vi "NistCSV2Cluster.vi"(8 "error in (no error)":errorcluster, 11 "NISTPath":path) -> (0 "error out":errorcluster, 2 "NISTData":T1 {"DataAnlysisArray"."TimeStamp" format="%^<%.3X\n%x>T"; "DUTDataArray"."Time Stamp" format="%^<%.3X\n%x>T"; "NIDataArray"."Time Stamp" format="%^<%.3X\n%x>T"})   [LabVIEW 2014]
uses:
  typedefs/NIData.ctl
  typedefs/PhasorRectangular.ctl
  typedefs/DUTData.ctl
  typedefs/NISTData.ctl
  typedefs/NIDataArray.ctl
  typedefs/NICalcAnalysis.ctl
  typedefs/CalcPhasorError.ctl
  <vilib>/Utility/miscctls.llb/LVDateTimeRec.ctl
  <vilib>/Utility/file.llb/Read From Spreadsheet File (string).vi
panel:
  in  "NICalcAnalysis":T6 {"TimeStamp" format="%^<%.3X\n%x>T"}
  in  "DUTDataCluster":T5 {"Time Stamp" format="%^<%.3X\n%x>T"}
  in  "NIDataCluster":T3 {"Time Stamp" format="%^<%.3X\n%x>T"}
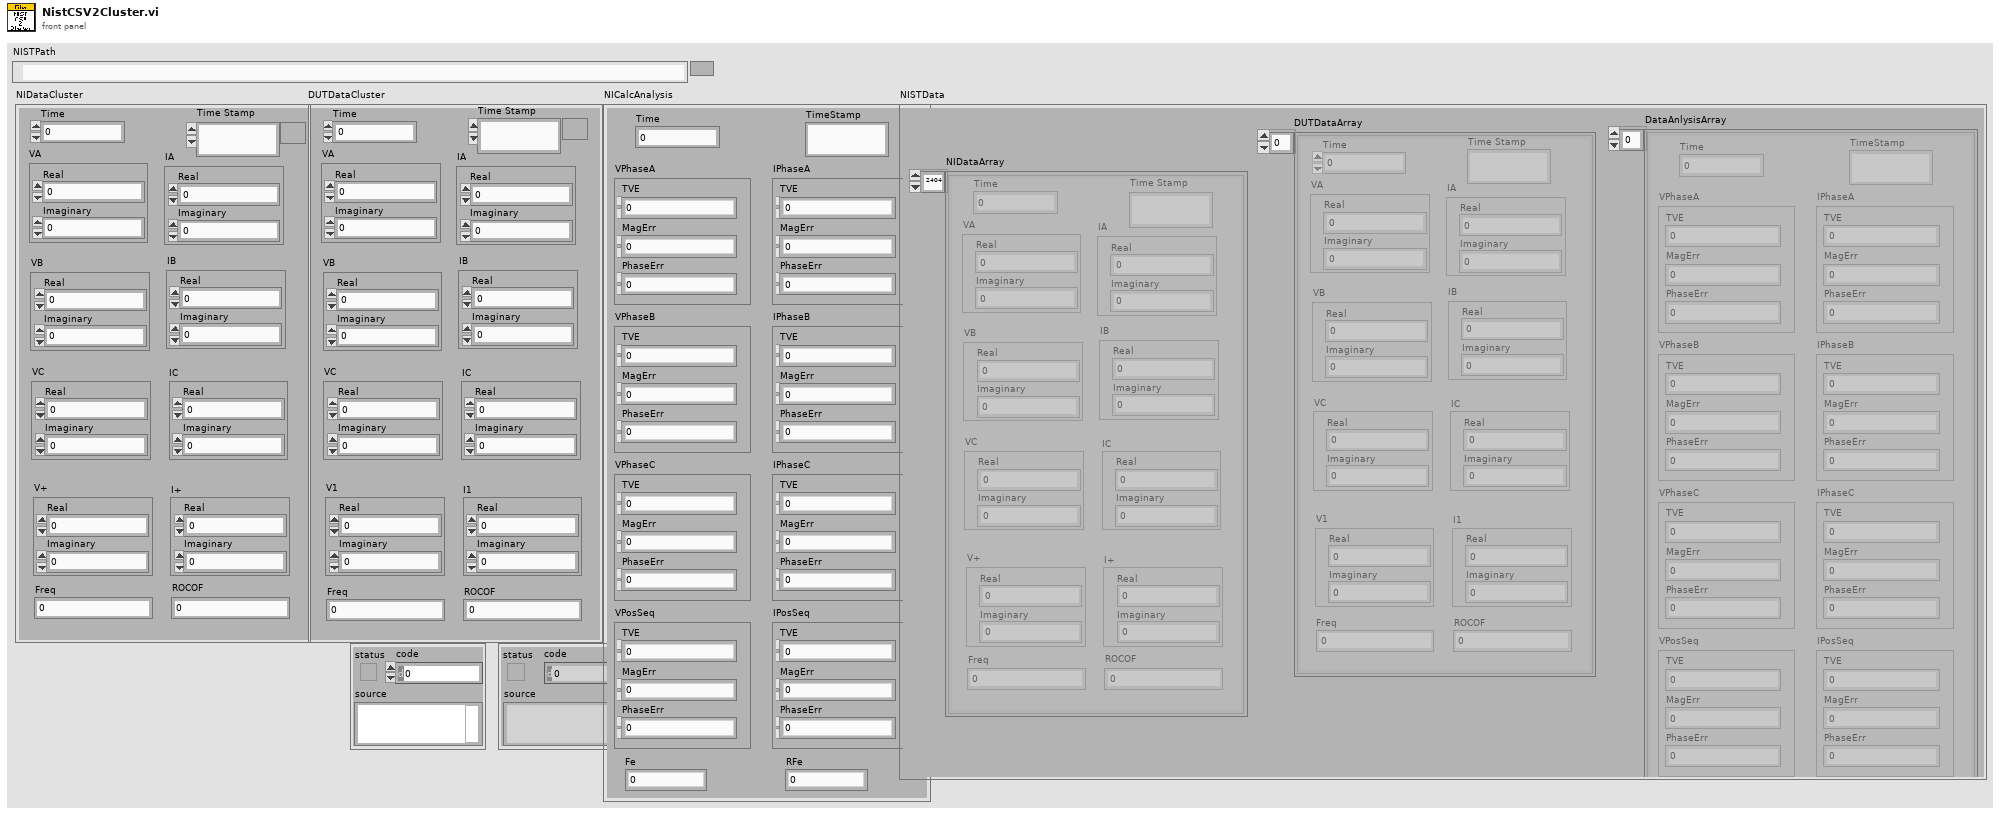
[diagram p1: front panel]
types:
  T1 = typedef "NISTData.ctl" = cluster{"NIDataArray":T2, "DUTDataArray":T5[], "DataAnlysisArray":T6[]}
  T2 = typedef "NIDataArray.ctl" = T3[]
  T3 = typedef "NIData.ctl" = cluster{"Time":dbl, "VA":T4, "VB":T4, "VC":T4, "V+":T4, "IA":T4, "IB":T4, "IC":T4, "I+":T4, "Freq":dbl, "ROCOF":dbl, "Time Stamp":timestamp}
  T4 = typedef "PhasorRectangular.ctl" = cluster{"Real":dbl, "Imaginary":dbl}
  T5 = typedef "DUTData.ctl" = cluster{"Time":dbl, "VA":T4, "VB":T4, "VC":T4, "V1":T4, "IA":T4, "IB":T4, "IC":T4, "I1":T4, "Freq":dbl, "ROCOF":dbl, "Time Stamp":timestamp}
  T6 = typedef "NICalcAnalysis.ctl" = cluster{"Time":dbl, "VPhaseA":T7, "IPhaseA":T7, "VPhaseB":T7, "IPhaseB":T7, "VPhaseC":T7, "IPhaseC":T7, "VPosSeq":T7, "IPosSeq":T7, "Fe":dbl, "RFe":dbl, "TimeStamp":timestamp}
  T7 = typedef "CalcPhasorError.ctl" = cluster{"TVE":dbl, "MagErr":dbl, "PhaseErr":dbl}
  T8 = typedef "LVDateTimeRec.ctl" = cluster{"fractional second":dbl, "second":i32, "minute":i32, "hour":i32, "day of month":i32, "month":i32, "year":i32, "day of week":i32, "day of year":i32, "DST":i32}
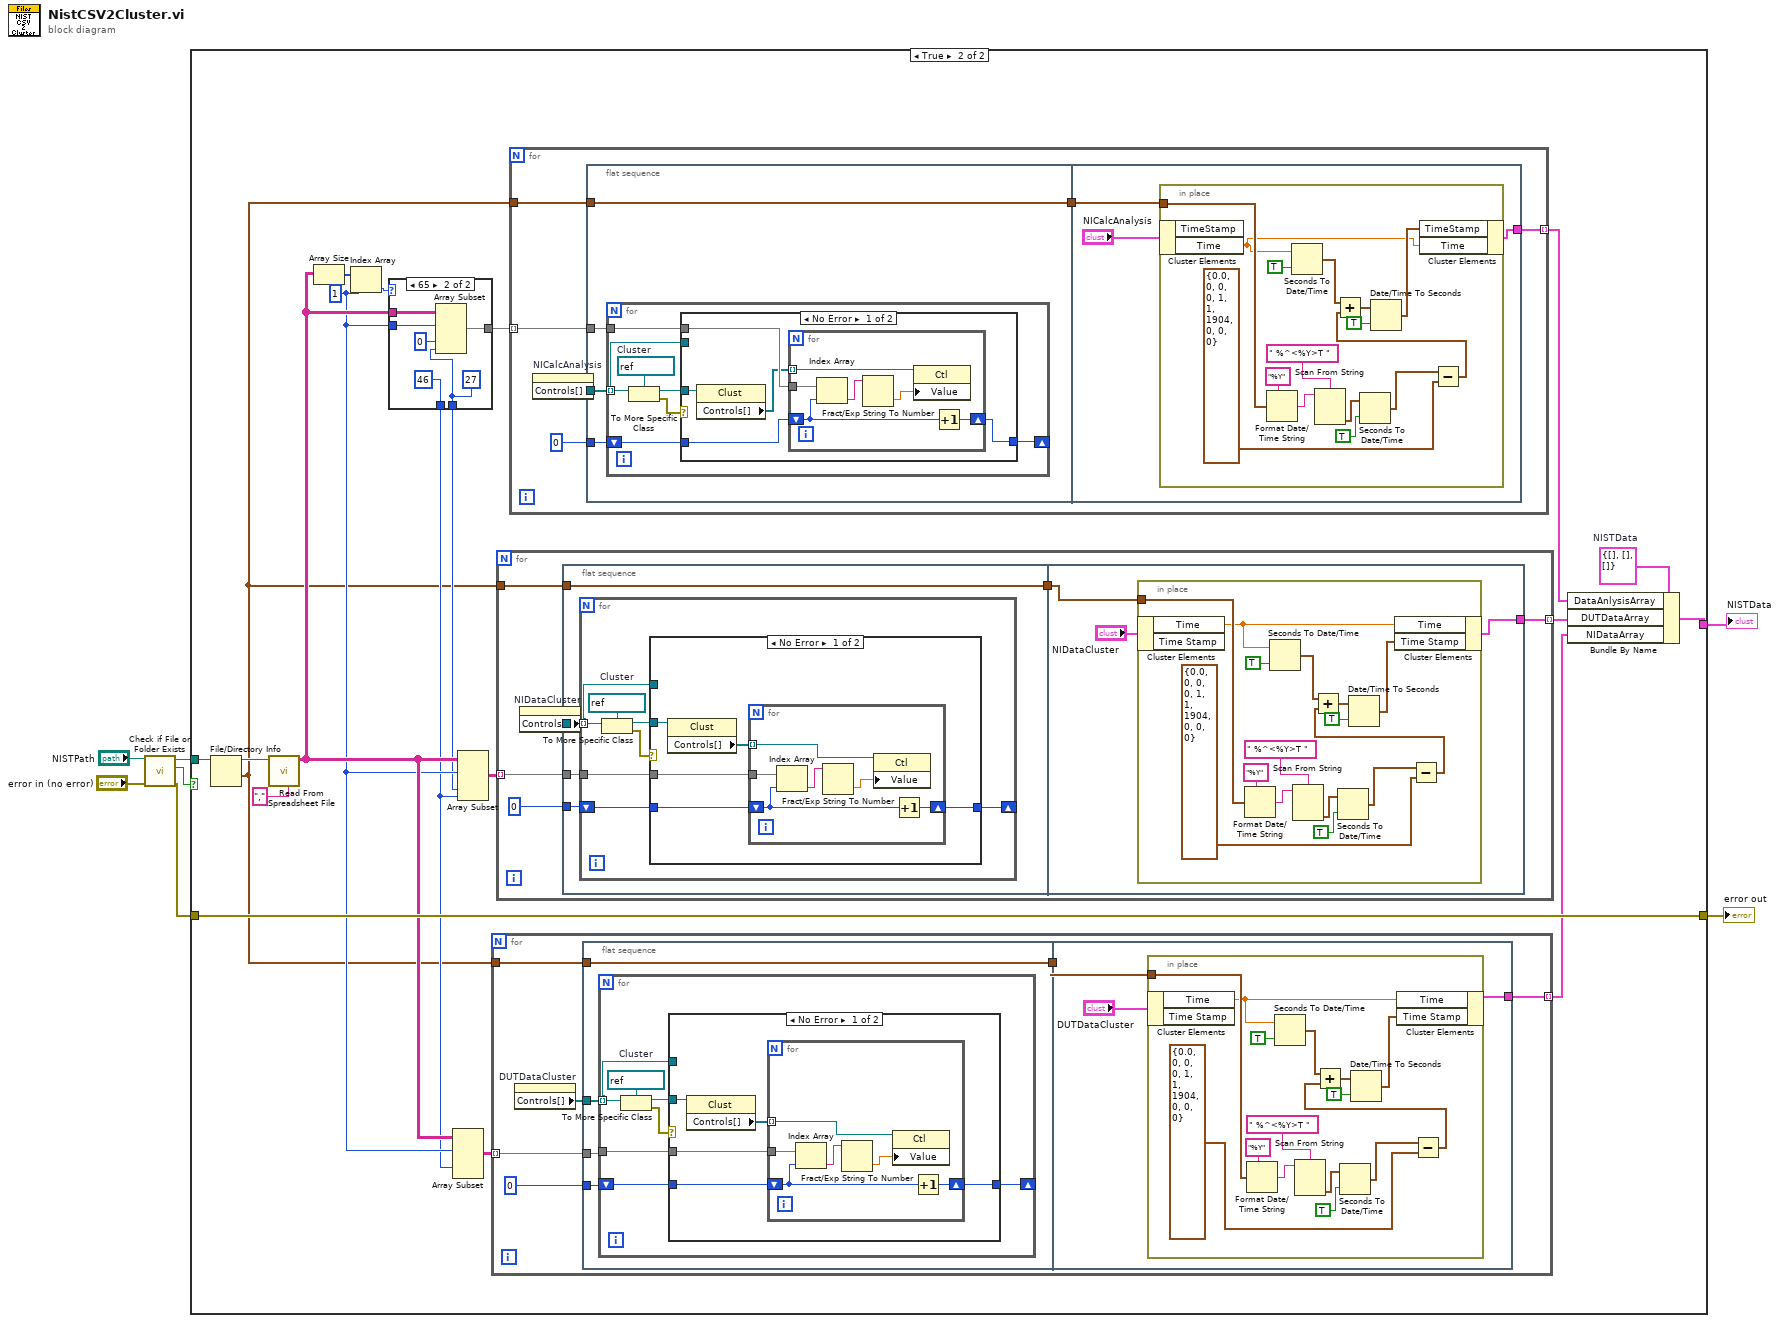
[diagram p0: block diagram]
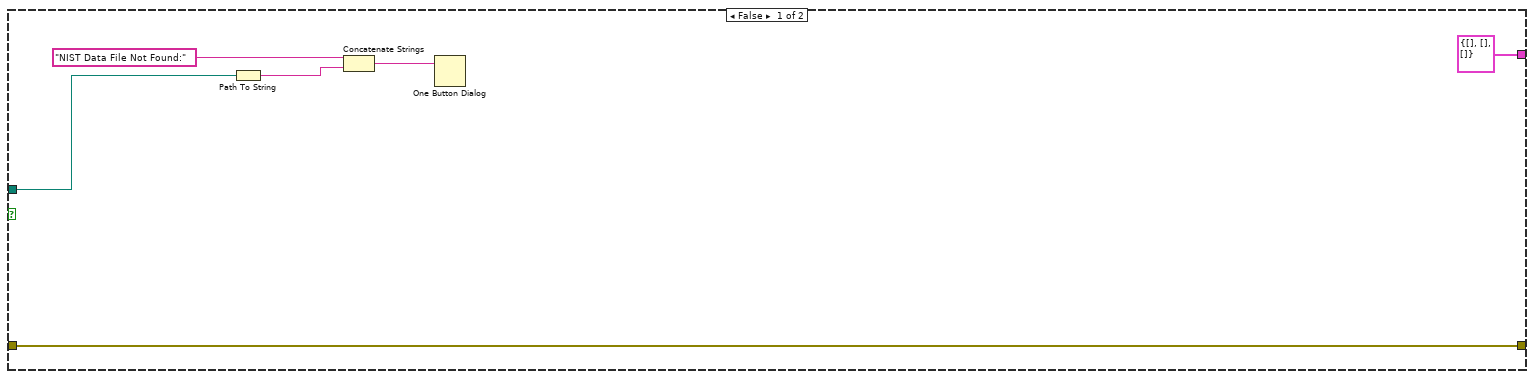
[diagram p2: hidden frame]
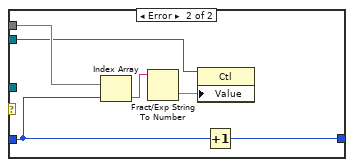
[diagram p3: hidden frame]
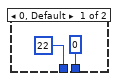
[diagram p4: hidden frame]
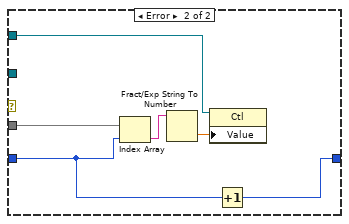
[diagram p5: hidden frame]
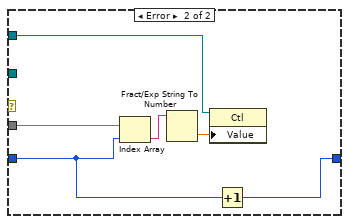
[diagram p6: hidden frame]
diagram:
  n1 = call <vilib>:"Check if File or Folder Exists.vi"("error in (no error)"="error in (no error)", "path"="NISTPath") -> ("error out"=w3:errorcluster, "file or folder exists?"=w4:bool, "dup path"=w5:path)  [unwired: 7 in]
  n2 = case shown="True" w4 {
    tunnel: w5 -> [w11 w32]
    tunnel: w3 -> [w9 w28]
    tunnel: [w9 w28] -> w2
    tunnel: [T1 {"NIDataArray"=[], "DUTDataArray"=[], "DataAnlysisArray"=[]} ("NISTData") w19] -> w1
    frame False {
      n3 = Path To String(path=w11) -> (string=w12:string)
      n4 = Concatenate Strings("NIST Data File Not Found:", w12) -> (w10:string)
      n5 = One Button Dialog(message=w10) -> ()  [unwired: 1 in, 1 out]
    }
    frame True {
      w22 = 1 ("index")
      w27 = T1 {"NIDataArray"=[], "DUTDataArray"=[], "DataAnlysisArray"=[]}  # NISTData
      n6 = File/Directory Info(path=w32) -> (path out=w26:path, last mod=w15:timestamp)  [unwired: 1 in, 5 out]
      n7 = call-poly <vilib>:"Read From Spreadsheet File.vi"("delimiter (\\t)"="," ("delimiter (\\t)"), "file path (dialog if empty)"=w26) -> ("all rows"=w23:string[][])  [unwired: 5 in, 4 out]
      n8 = Array Size(array=w23) -> (size(s)=w25:i32[])
      n9 = Index Array(array=w25, index=w22) -> (element=w24:i32)
      n10 = case shown="65" w24 {
        tunnel: w23 -> [_ w92]
        tunnel: w22 -> [_ w91]
        tunnel: [0 ("index") w88] -> w21
        tunnel: [22 ("length") 46 ("length")] -> w20
        tunnel: [_ w87] -> w16
        frame 0, Default {
        }
        frame 65 {
          w88 = 27 ("index")
          n11 = Array Subset(array=w92, index (row)=w91, index (col)=0 ("index"), length (col)=w88) -> (w87:string[][])  [unwired: 1 in]
        }
      }
      n12 = Array Subset(array=w23, index (row)=w22, index (col)=w20) -> (w29:string[][])  [unwired: 2 in]
      n13 = Array Subset(array=w23, index (row)=w22, index (col)=w21, length (col)=w20) -> (w30:string[][])  [unwired: 1 in]
      n14 = for {
        tunnel: w29 -> [w98] mode=indexing
        tunnel: [w93] -> w17 mode=indexing
        tunnel: w15 -> [w95]
        n15 = property on="DUTDataCluster" class="Clust (strict)"() -> ("Controls[]"=w96:refnum<vi>[])  [unwired: 2 in, 2 out]
        n16 = flat-sequence {
          tunnel: w98 -> [w102]
          tunnel: 0 ("index") -> [w101]
          tunnel: w96 -> [w100]
          tunnel: w95 -> [w99]
          tunnel: [w99] -> w94
          tunnel: w94 -> [w128]
          tunnel: [w127] -> w93
          frame #0 {
            n17 = for {
              tunnel: w100 -> [w103] mode=indexing
              tunnel: w102 -> [w106]
              shift-right: [w104] -> _
              shift-left: w101 -> [w105]
              w109 = refnum<vi> refnum  # Cluster
              n18 = To More Specific Class(target class=w109, reference=w103) -> (specific class reference=w107:refnum<vi>, error out=w108:errorcluster)  [unwired: 1 in]
              n19 = case shown="No Error" w108 {
                tunnel: w107 -> [w114 _]
                tunnel: w106 -> [w112 w126]
                tunnel: w105 -> [w111 w125]
                tunnel: [w110 w124] -> w104
                tunnel: w103 -> [_ w121]
                frame No Error {
                  n20 = property class="Clust"(reference=w114) -> ("Controls[]"=w113:refnum<vi>[])  [unwired: 1 in, 2 out]
                  n21 = for {
                    tunnel: w113 -> [w117] mode=indexing
                    tunnel: w112 -> [w120]
                    shift-right: [w115] -> w110
                    shift-left: w111 -> [w119]
                    n22 = Index Array(array=w120, index=w119) -> (element=w118:string)
                    n23 = Fract/Exp String To Number(string=w118) -> (number=w116:dbl)  [unwired: 3 in, 1 out]
                    n24 = property class="Ctl"(reference=w117, "Value"=w116) -> ()  [unwired: 1 in, 2 out]
                    n25 = Increment(x=w119) -> (x+1=w115:i32)
                  }
                }
                frame Error {
                  n26 = Index Array(array=w126, index=w125) -> (element=w123:string)
                  n27 = Fract/Exp String To Number(string=w123) -> (number=w122:dbl)  [unwired: 3 in, 1 out]
                  n28 = property class="Ctl"(reference=w121, "Value"=w122) -> ()  [unwired: 1 in, 2 out]
                  n29 = Increment(x=w125) -> (x+1=w124:i32)
                }
              }
            }
          }
          frame #1 {
            n30 = in-place {
              in-place-border: w128 -> [w144]
              n31 = in-place-cluster #1("DUTDataCluster") -> ("Time"=w140:dbl)  [unwired: 1 out]
              n32 = Format Date/Time String(time format string (%c)="%Y", seconds (now)=w144) -> (date/time string=w141:string)  [unwired: 1 in]
              n33 = Seconds To Date/Time(time stamp (now)=w140, to UTC (F)=TRUE) -> (date time rec=w138:T8)
              n34 = Scan From String(format string=" %^<%Y>T ", input string=w141) -> (output 1=w139:timestamp)  [unwired: 3 in, 3 out]
              n35 = Seconds To Date/Time(time stamp (now)=w139, to UTC (F)=TRUE ("is UTC (F)")) -> (date time rec=w135:T8)
              n36 = Subtract(x=w135, y=T8 {"fractional second"=0.0, "second"=0, "minute"=0, "hour"=0, "day of month"=1, "month"=1, "year"=1904, "day of week"=0, "day of year"=0, "DST"=0}) -> (x-y=w134:T8)
              n37 = Add(x=w138, y=w134) -> (x+y=w137:T8)
              n38 = Date/Time To Seconds(1:TRUE ("is UTC (F)"), 2:w137) -> (0:w136:timestamp)
              n39 = in-place-cluster #1("Time"=w140, "Time Stamp"=w136) -> (w127:T5)
            }
          }
        }
      }
      n40 = for {
        tunnel: w30 -> [w150] mode=indexing
        tunnel: [w145] -> w18 mode=indexing
        tunnel: w15 -> [w146]
        n41 = property on="NIDataCluster" class="Clust (strict)"() -> ("Controls[]"=w148:refnum<vi>[])  [unwired: 2 in, 2 out]
        n42 = flat-sequence {
          tunnel: w150 -> [w154]
          tunnel: 0 ("index") -> [w153]
          tunnel: w148 -> [w152]
          tunnel: [w151] -> w147
          tunnel: w146 -> [w151]
          tunnel: w147 -> [w180]
          tunnel: [w179] -> w145
          frame #0 {
            n43 = for {
              tunnel: w152 -> [w155] mode=indexing
              tunnel: w154 -> [w158]
              shift-right: [w156] -> _
              shift-left: w153 -> [w157]
              w161 = refnum<vi> refnum  # Cluster
              n44 = To More Specific Class(target class=w161, reference=w155) -> (specific class reference=w159:refnum<vi>, error out=w160:errorcluster)  [unwired: 1 in]
              n45 = case shown="No Error" w160 {
                tunnel: w159 -> [w166 _]
                tunnel: w158 -> [w164 w178]
                tunnel: w157 -> [w163 w177]
                tunnel: [w162 w176] -> w156
                tunnel: w155 -> [_ w173]
                frame No Error {
                  n46 = property class="Clust"(reference=w166) -> ("Controls[]"=w165:refnum<vi>[])  [unwired: 1 in, 2 out]
                  n47 = for {
                    tunnel: w165 -> [w169] mode=indexing
                    tunnel: w164 -> [w172]
                    shift-right: [w167] -> w162
                    shift-left: w163 -> [w171]
                    n48 = Index Array(array=w172, index=w171) -> (element=w170:string)
                    n49 = Fract/Exp String To Number(string=w170) -> (number=w168:dbl)  [unwired: 3 in, 1 out]
                    n50 = property class="Ctl"(reference=w169, "Value"=w168) -> ()  [unwired: 1 in, 2 out]
                    n51 = Increment(x=w171) -> (x+1=w167:i32)
                  }
                }
                frame Error {
                  n52 = Index Array(array=w178, index=w177) -> (element=w175:string)
                  n53 = Fract/Exp String To Number(string=w175) -> (number=w174:dbl)  [unwired: 3 in, 1 out]
                  n54 = property class="Ctl"(reference=w173, "Value"=w174) -> ()  [unwired: 1 in, 2 out]
                  n55 = Increment(x=w177) -> (x+1=w176:i32)
                }
              }
            }
          }
          frame #1 {
            n56 = in-place {
              in-place-border: w180 -> [w196]
              n57 = in-place-cluster #2("NIDataCluster") -> ("Time"=w192:dbl)  [unwired: 1 out]
              n58 = Format Date/Time String(time format string (%c)="%Y", seconds (now)=w196) -> (date/time string=w193:string)  [unwired: 1 in]
              n59 = Seconds To Date/Time(time stamp (now)=w192, to UTC (F)=TRUE) -> (date time rec=w190:T8)
              n60 = Scan From String(format string=" %^<%Y>T ", input string=w193) -> (output 1=w191:timestamp)  [unwired: 3 in, 3 out]
              n61 = Seconds To Date/Time(time stamp (now)=w191, to UTC (F)=TRUE) -> (date time rec=w187:T8)
              n62 = Subtract(x=w187, y=T8 {"fractional second"=0.0, "second"=0, "minute"=0, "hour"=0, "day of month"=1, "month"=1, "year"=1904, "day of week"=0, "day of year"=0, "DST"=0}) -> (x-y=w184:T8)
              n63 = Add(x=w190, y=w184) -> (x+y=w189:T8)
              n64 = Date/Time To Seconds(1:TRUE ("is UTC (F)"), 2:w189) -> (0:w188:timestamp)
              n65 = in-place-cluster #2("Time"=w192, "Time Stamp"=w188) -> (w179:T3)
            }
          }
        }
      }
      n66 = for {
        tunnel: w16 -> [w37] mode=indexing
        tunnel: w15 -> [w36]
        tunnel: [w33] -> w14 mode=indexing
        n67 = property on="NICalcAnalysis" class="Clust (strict)"() -> ("Controls[]"=w34:refnum<vi>[])  [unwired: 2 in, 2 out]
        n68 = flat-sequence {
          tunnel: w34 -> [w42]
          tunnel: 0 ("index") -> [w41]
          tunnel: w37 -> [w40]
          tunnel: w36 -> [w39]
          tunnel: [w39] -> w35
          tunnel: w35 -> [w68]
          tunnel: [w67] -> w33
          frame #0 {
            n69 = for {
              tunnel: w42 -> [w43] mode=indexing
              shift-right: [w44] -> _
              shift-left: w41 -> [w46]
              tunnel: w40 -> [w45]
              w49 = refnum<vi> refnum  # Cluster
              n70 = To More Specific Class(target class=w49, reference=w43) -> (specific class reference=w47:refnum<vi>, error out=w48:errorcluster)  [unwired: 1 in]
              n71 = case shown="No Error" w48 {
                tunnel: w47 -> [w54 _]
                tunnel: w46 -> [w53 w63]
                tunnel: w45 -> [w51 w64]
                tunnel: [w52 w62] -> w44
                tunnel: w43 -> [_ w61]
                frame No Error {
                  n72 = property class="Clust"(reference=w54) -> ("Controls[]"=w50:refnum<vi>[])  [unwired: 1 in, 2 out]
                  n73 = for {
                    tunnel: w50 -> [w57] mode=indexing
                    tunnel: w51 -> [w60]
                    shift-right: [w55] -> w52
                    shift-left: w53 -> [w59]
                    n74 = Index Array(array=w60, index=w59) -> (element=w58:string)
                    n75 = Fract/Exp String To Number(string=w58) -> (number=w56:dbl)  [unwired: 3 in, 1 out]
                    n76 = property class="Ctl"(reference=w57, "Value"=w56) -> ()  [unwired: 1 in, 2 out]
                    n77 = Increment(x=w59) -> (x+1=w55:i32)
                  }
                }
                frame Error {
                  n78 = Index Array(array=w64, index=w63) -> (element=w65:string)
                  n79 = Fract/Exp String To Number(string=w65) -> (number=w66:dbl)  [unwired: 3 in, 1 out]
                  n80 = property class="Ctl"(reference=w61, "Value"=w66) -> ()  [unwired: 1 in, 2 out]
                  n81 = Increment(x=w63) -> (x+1=w62:i32)
                }
              }
            }
          }
          frame #1 {
            n82 = in-place {
              in-place-border: w68 -> [w84]
              n83 = in-place-cluster #3("NICalcAnalysis") -> ("Time"=w70:dbl)  [unwired: 1 out]
              n84 = Format Date/Time String(time format string (%c)="%Y", seconds (now)=w84) -> (date/time string=w81:string)  [unwired: 1 in]
              n85 = Seconds To Date/Time(time stamp (now)=w70, to UTC (F)=TRUE) -> (date time rec=w79:T8)
              n86 = Scan From String(format string=" %^<%Y>T ", input string=w81) -> (output 1=w80:timestamp)  [unwired: 3 in, 3 out]
              n87 = Seconds To Date/Time(time stamp (now)=w80, to UTC (F)=TRUE) -> (date time rec=w77:T8)
              n88 = Subtract(x=w77, y=T8 {"fractional second"=0.0, "second"=0, "minute"=0, "hour"=0, "day of month"=1, "month"=1, "year"=1904, "day of week"=0, "day of year"=0, "DST"=0}) -> (x-y=w74:T8)
              n89 = Add(x=w79, y=w74) -> (x+y=w78:T8)
              n90 = Date/Time To Seconds(1:TRUE ("is UTC (F)"), 2:w78) -> (0:w71:timestamp)
              n91 = in-place-cluster #3("TimeStamp"=w71, "Time"=w70) -> (w67:T6)
            }
          }
        }
      }
      n92 = Bundle By Name(cluster=w27, "DataAnlysisArray"=w14, "DUTDataArray"=w18, "NIDataArray"=w17) -> (w19:T1)
    }
  }
  "error out" <- w2
  "NISTData" <- w1
